vi "Setup for new units-Hybrid.vi"(0 "SC Current [kA]":dbl format="%.5f", 3 "error in (no error)":errorcluster) -> (1 "Field Setpoint Caption":string, 2 "Field Slew Rate Caption":string, 4 "Field Range":T1 {"Increment" format="%.2f"; "Maximum" format="%.2f"; "Minimum" format="%.2f"}, 5 "Current Setpoint Caption":string, 6 "Current Slew Rate Caption":string, 7 "Current Range":T1 {"Increment" format="%.2f"; "Maximum" format="%.2f"; "Minimum" format="%.2f"})   [LabVIEW 2019]
uses:
  PS Comm Globals.vi
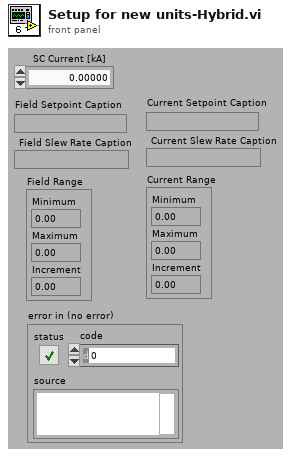
[diagram p1: front panel]
types:
  T1 = cluster{"Minimum":dbl, "Maximum":dbl, "Increment":dbl}
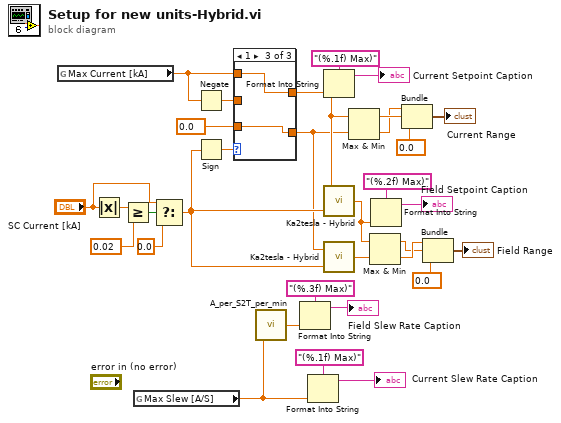
[diagram p0: block diagram]
diagram:
  n1 = global read "PS Comm Globals.vi" "Max Current [kA]"() -> (w2:dbl)
  n2 = Absolute Value(x="SC Current [kA]") -> (abs(x)=w9:dbl)
  n3 = Greater Or Equal?(x=w9, y=0.02) -> (x >= y?=w10:bool)
  n4 = global read "PS Comm Globals.vi" "Max Slew [A/S]"() -> (w23:dbl)
  n5 = Select(t="SC Current [kA]", s=w10, f=0.0) -> (s? t:f=w5:dbl)
  n6 = Negate(x=w2) -> (-x=w1:dbl)
  n7 = Sign(1:w5) -> (0:w18:dbl)
  n8 = case shown="1" w18 {
    tunnel: w2 -> [_ w36 w38]
    tunnel: [w33 w36 w38] -> w13
    tunnel: [w34 w35 w37] -> w4
    tunnel: 0.0 -> [w34 _ w37]
    tunnel: w1 -> [w33 w35 _]
    frame -1 {
    }
    frame 0, Default {
    }
    frame 1 {
    }
  }
  n9 = call "A_per_S2T_per_min.vi"("A/sec"=w23) -> ("T/min"=w28:dbl)
  n10 = Format Into String(format string="(%.3f) Max)", w28) -> (resulting string=→"Field Slew Rate Caption":string)  [unwired: 2 in, 1 out]
  n11 = Format Into String(format string="(%.1f) Max)", w23) -> (resulting string=→"Current Slew Rate Caption":string)  [unwired: 2 in, 1 out]
  n12 = Format Into String(format string="(%.1f) Max)", w13) -> (resulting string=→"Current Setpoint Caption":string)  [unwired: 2 in, 1 out]
  n13 = call "Ka2tesla - Hybrid.vi"("SC Current [kA]"=w5, "Current [KA]"=w13) -> ("Field"=w16:dbl)
  n14 = call "Ka2tesla - Hybrid.vi"("SC Current [kA]"=w5, "Current [KA]"=w4) -> ("Field"=w19:dbl)
  n15 = Max & Min(x=w13, y=w4) -> (max(x,y)=w14:dbl, min(x,y)=w11:dbl)
  n16 = Max & Min(x=w16, y=w19) -> (max(x,y)=w15:dbl, min(x,y)=w17:dbl)
  n17 = Format Into String(format string="(%.2f) Max)", w16) -> (resulting string=→"Field Setpoint Caption":string)  [unwired: 2 in, 1 out]
  n18 = Bundle(w11, w14, 0.0) -> (→"Current Range":cluster{dbl, dbl, dbl})  [unwired: 1 in]
  n19 = Bundle(w17, w15, 0.0) -> (→"Field Range":cluster{dbl, dbl, dbl})  [unwired: 1 in]
